vi "Set Timestamp.vi"(0 "image in":refnum<class "MSC Image.lvclass">, 1 "Time Stamp":timestamp, 5 "error in (no error)":errorcluster) -> (14 "image out":refnum<class "MSC Image.lvclass">, 19 "error out":errorcluster)   [LabVIEW 2016, in "MSC Image.lvclass"]
doc: "Sets the image timestamp. If the input is unwired, it is set to the current timestamp."
uses:
  MSC Image.lvclass
  MSC Image.lvclass/MSC Image.ctl
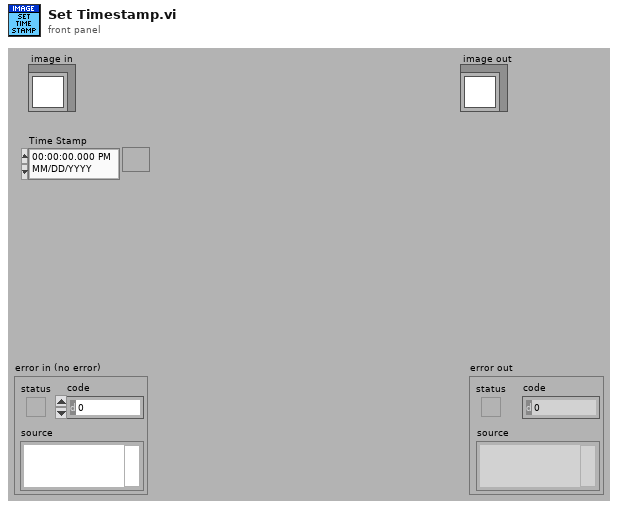
[diagram p1: front panel]
types:
  T1 = typedef "Image.ctl" = cluster{"Pointer":u64, "Size":T2, "Image Type":T3, "Time Stamp":timestamp, "Variant":variant}
  T2 = typedef "Size.ctl" = cluster{"Cols":i32, "Rows":i32}
  T3 = typedef "Image Type.ctl" = i32
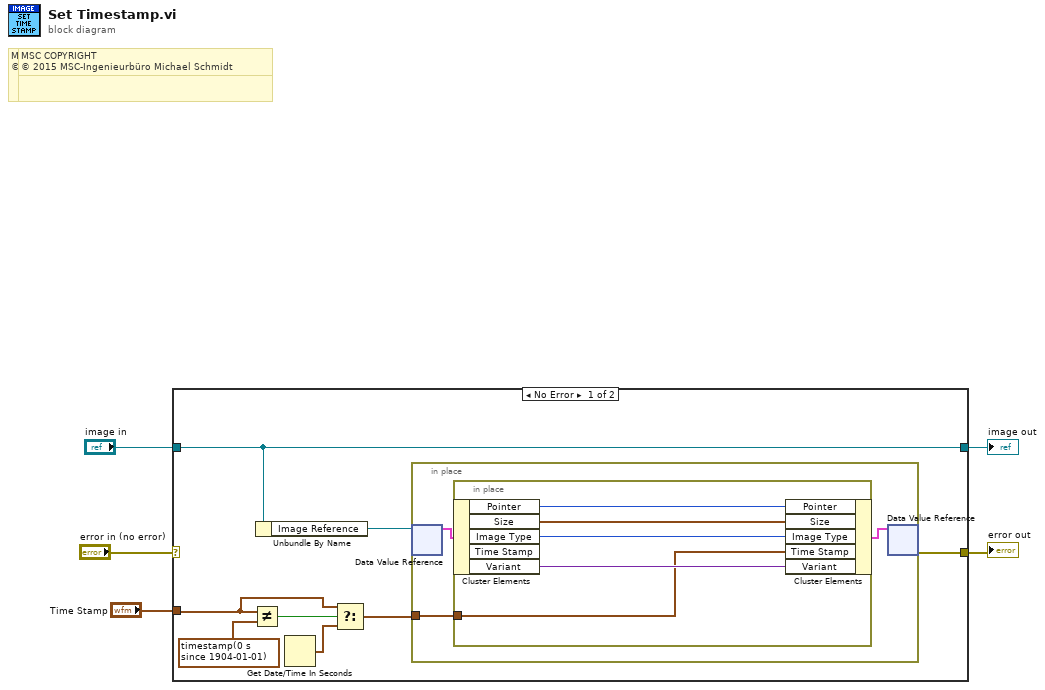
[diagram p0: block diagram]
diagram:
  # "MSC COPYRIGHT\n© 2016 MSC-Ingenieurbüro Michael Schmidt"
  # "MSC COPYRIGHT\n© 2016 MSC-Ingenieurbüro Michael Schmidt"
  # "MSC COPYRIGHT\n© 2015 MSC-Ingenieurbüro Michael Schmidt"
  # "MSC COPYRIGHT\n© 2015 MSC-Ingenieurbüro Michael Schmidt"
  n1 = case shown="No Error" "error in (no error)" {
    selector: "error in (no error)" -> [_ w23]
    tunnel: [w11 w23] -> w4
    tunnel: [w13 w22] -> w2
    tunnel: "image in" -> [w13 w22]
    tunnel: "Time Stamp" -> [w8 _]
    frame No Error {
      n2 = Not Equal?(x=w8, y=timestamp(0 s since 1904-01-01)) -> (x != y?=w9:bool)
      n3 = Unbundle By Name(w13) -> ("Image Reference"=w12:refnum<data-value>)
      n4 = Get Date/Time In Seconds() -> (seconds since 1Jan1904=w7:timestamp)
      n5 = Select(t=w8, s=w9, f=w7) -> (s? t:f=w6:timestamp)
      n6 = in-place {
        in-place-border: w6 -> [w14]
        n7 = in-place-dvr #1(w12) -> (w15:T1)  [unwired: 1 out]
        n8 = in-place {
          in-place-border: w14 -> [w17]
          n9 = in-place-cluster #2(w15) -> ("Pointer"=w21:u64, "Size"=w20:T2, "Image Type"=w19:T3, "Variant"=w18:variant)  [unwired: 1 out]
          n10 = in-place-cluster #2("Pointer"=w21, "Size"=w20, "Image Type"=w19, "Time Stamp"=w17, "Variant"=w18) -> (w16:T1)
        }
        n11 = in-place-dvr #1(w16) -> (w11:errorcluster)  [unwired: 1 out]
      }
    }
    frame Error {
    }
  }
  "error out" <- w4
  "image out" <- w2
